vi "Refresh_Image_by_Copying_Fresh_One-1.vi"(4 "[IN] Image Type":T3 items=["Grayscale (U8)", "Grayscale (I16)", "Grayscale (SGL)", "Complex (CSG)", "RGB (U32)", "HSL (U32)", "RGB (U64)", "Grayscale (U16)"], 5 "[IN] Unique ID\n(# of Event)":string, 6 "error IN":errorcluster, 7 "Frame Number":u32, 8 "[IN] Preinitialized Image":T1, 9 "[IN] AVI Refnum":T2) -> (0 "error OUT":errorcluster, 2 "[OUT] Frame":T1, 3 "[OUT] AVI Refnum":T2)   [LabVIEW 2013]
doc: "Subprogram refreshes the image by copying new frame from video to destination image \nInitialized image is disposed after it for preventing using too much images\nOperation of copying refresh one preinitialized image for further processing / visualization"
uses:
  <vilib>/vision/Avi.llb/IMAQ AVI2 Refnum.ctl
  <vilib>/vision/Image Controls.llb/IMAQ Image.ctl
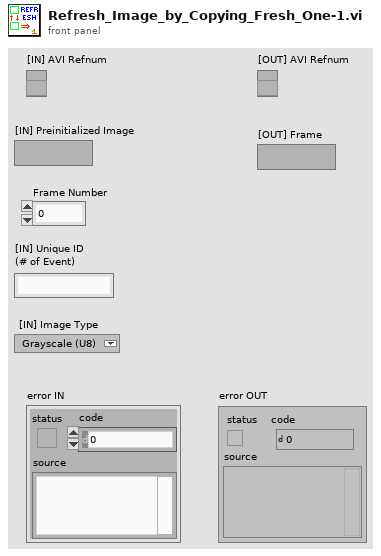
[diagram p1: front panel]
types:
  T1 = typedef "IMAQ Image.ctl" = refnum<image>
  T2 = typedef "IMAQ AVI2 Refnum.ctl" = refnum<k20>
  T3 = typedef "Image Type" = u32
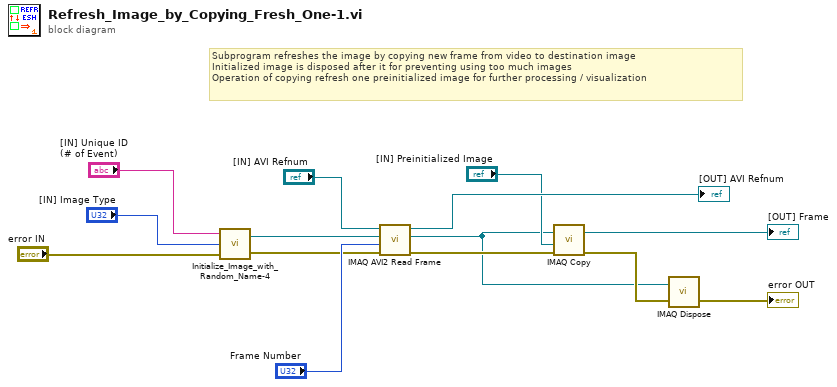
[diagram p0: block diagram]
diagram:
  # "Subprogram refreshes the image by copying new frame from video to destination image \nInitialized image is disposed after it for preventing using too much images\nOperation of copying refresh one preinitialized image for further processing / visualization"
  n1 = call "Initialize_Image_with_Random_Name-4.vi"("error IN"="error IN", "Image Type"="[IN] Image Type", "Unique ID"="[IN] Unique ID\n(# of Event)") -> ("error OUT"=w8:errorcluster, "[OUT] New Image"=w10:T1)
  n2 = call "IMAQ AVI2 Read Frame"("error in (no error)"=w8, "Frame Number"="Frame Number", "Image"=w10, "AVI Refnum"="[IN] AVI Refnum") -> ("error out"=w6:errorcluster, "Image Out"=w2:T1, "AVI Refnum (duplicate)"=→"[OUT] AVI Refnum":T2)  [unwired: 5 in]
  n3 = call "IMAQ Copy"("error in (no error)"=w6, "Image Dst"="[IN] Preinitialized Image", "Image Src"=w2) -> ("error out"=w3:errorcluster, "Image Dst Out"=→"[OUT] Frame":T1)  [unwired: 3 in]
  n4 = call "IMAQ Dispose"("Image"=w2, "error in (no error)"=w3) -> ("error out"=→"error OUT":errorcluster)  [unwired: 4 in]
